vi "LVClass_WavefrontCorrector ctor.vi"(0 "WavefrontCorrector in":refnum<class "WavefrontCorrector.lvclass">, 5 "PathToWavefrontCorrectorSetupFile":path, 11 "error in (no error)":errorcluster) -> (4 "WavefrontCorrector out":refnum<class "WavefrontCorrector.lvclass">, 15 "error out":errorcluster)   [LabVIEW 2020, in "WavefrontCorrector.lvclass"]
doc: "WavefrontCorrector constructor.\n\n--------------------------------------------------------------------------------\n\n<B>correctorIn </B> : Constant Pointer to WavefrontCorrector object.\n<B>correctorOut </B> : Constant Pointer to WavefrontCorrector object.\n<B>config_file_path </B> : Absolute path to Wavefront corrector configuration file.\n<B>ErrorIn </B> : Error\n<B>ErrorOut </B> : Error\n\n--------------------------------------------------------------------------------"
uses:
  WavefrontCorrector.lvclass
  WavefrontCorrectorSet.lvclass
  Wavefront Corrector states - ONE.ctl
  WavefrontCorrector.lvclass/WavefrontCorrector.ctl
  Handle creation.ctl
  LVClass_WavefrontCorrectorSet Read AllWavefrontCorrectorParametersProperties.vi
  LVClass_WavefrontCorrectorSet Read AllWavefrontCorrectorParameters.vi
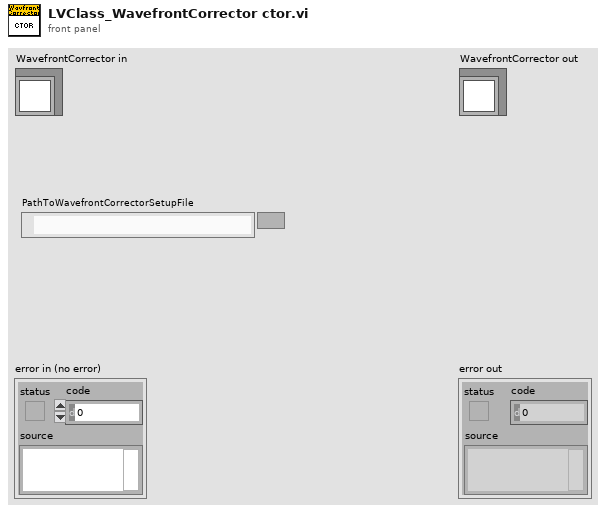
[diagram p1: front panel]
types:
  T1 = typedef "Wavefront Corrector states - ONE.ctl" = cluster{"Max":sgl, "Min":sgl, "Validity":enum16{"valid", "fixed", "invalid"}, "Fixed_Position":sgl}
  T2 = typedef "Handle creation.ctl" = enum16{"By ctor", "By write function"}
  T3 = typedef "WavefrontCorrectorSpecifications.ctl" = cluster{"Mirror name":string, "Plugin name":string, "Serial number":string, "Revision":string, "Number of commands":i32, "Sleep after command apply (ms)":i32, "Has internal memory ?":bool}
  T4 = typedef "ParameterID.ctl" = cluster{"Name":string, "Type":T5, "Authorization":T6, "OnFlyAuthorization":T7, "StringDefault":string, "Default":dbl, "Min":dbl, "Max":dbl, "Boolean":bool, "StringParameterList":string[]}
  T5 = typedef "CameraParameters_Type.ctl" = enum16{"Integer", "Real", "String", "Boolean"}
  T6 = typedef "CameraParameters_Authorization.ctl" = enum16{"Disable", "Gettable", "Settable - Gettable"}
  T7 = typedef "CameraParameters_OnFlyAuthorization.ctl" = enum16{"None", "Gettable", "Settable", "Settable - Gettable"}
  T8 = typedef "CameraParametersSetup.ctl" = cluster{"Name":string, "Type":T5, "Value":dbl, "BooleanValue":bool, "StringValue":string}
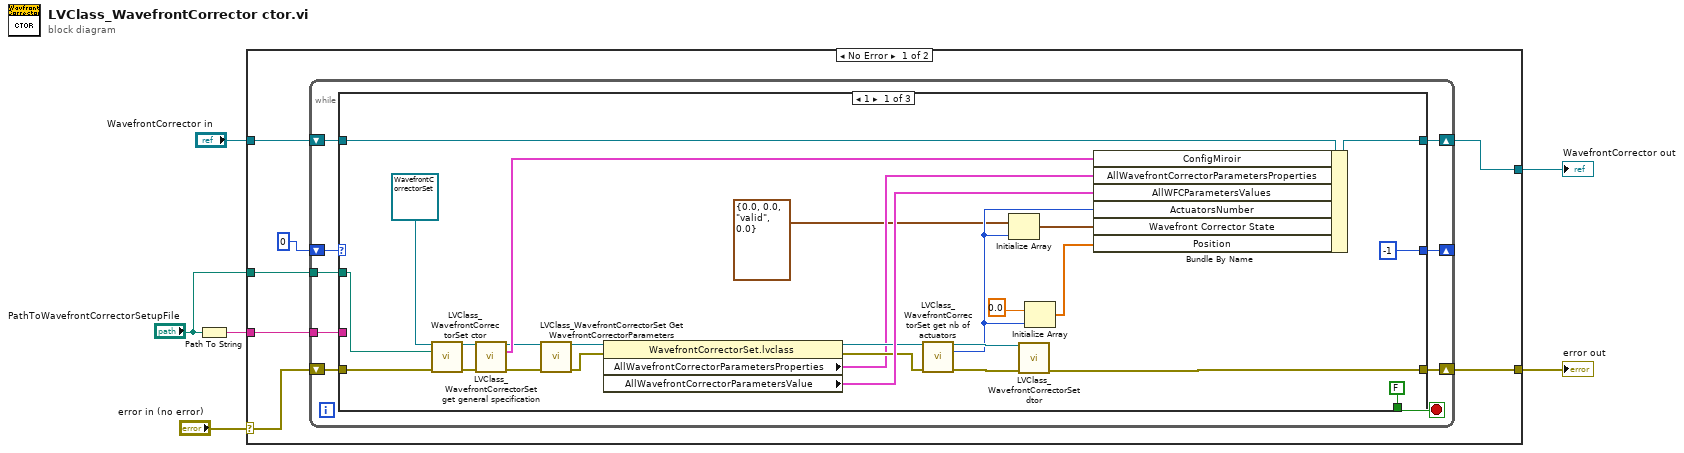
[diagram p0: block diagram]
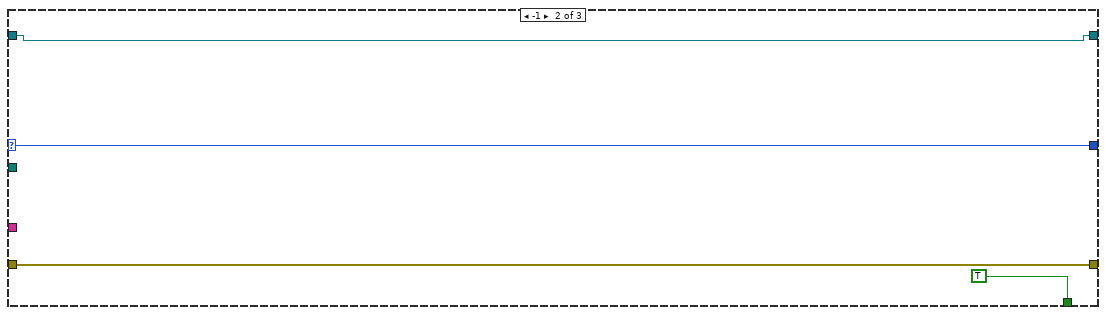
[diagram p2: hidden frame]
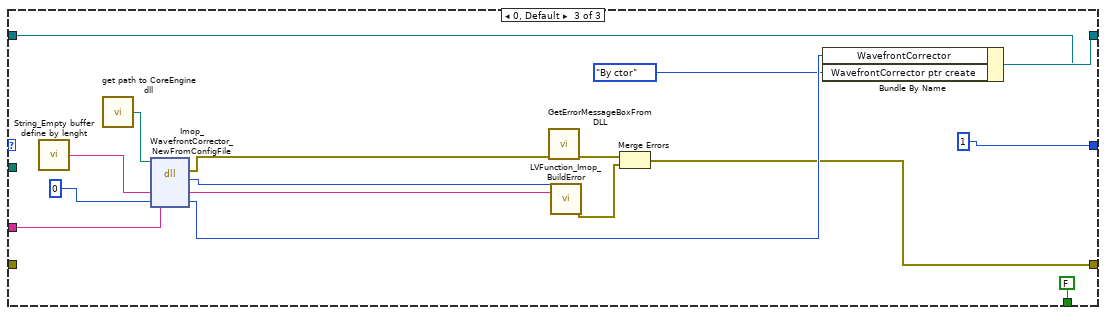
[diagram p3: hidden frame]
diagram:
  n1 = Path To String(path="PathToWavefrontCorrectorSetupFile") -> (string=w6:string)
  n2 = case shown="No Error" "error in (no error)" {
    selector: "error in (no error)" -> [w8 w70]
    tunnel: [w7 w70] -> w3
    tunnel: [w12 w69] -> w2
    tunnel: "WavefrontCorrector in" -> [w13 w69]
    tunnel: w6 -> [w11 _]
    tunnel: "PathToWavefrontCorrectorSetupFile" -> [w9 _]
    frame No Error {
      n3 = while {
        tunnel: w11 -> [w21]
        shift-right: [w19] -> _
        shift-left: 0 -> [w20]
        tunnel: w9 -> [w18]
        shift-right: [w15] -> w7
        shift-left: w8 -> [w16]
        shift-right: [w22] -> w12
        shift-left: w13 -> [w17]
        stop <- w14 stop-if-true
        n4 = case shown="1" w20 {
          selector: w20 -> [_ w52 _]
          tunnel: [w36 w49 w60] -> w22
          tunnel: [w37 w51 w57] -> w15
          tunnel: w21 -> [_ _ w56]
          tunnel: [-1 w52 1] -> w19
          tunnel: w18 -> [w46 _ _]
          tunnel: w17 -> [w45 w49 w53]
          tunnel: w16 -> [w42 w51 _]
          tunnel: [FALSE TRUE FALSE] -> w14
          frame 1 {
            n5 = call "LVClass_WavefrontCorrectorSet ctor.vi"("WavefrontCorrectorSet in"=refnum<class "WavefrontCorrectorSet.lvclass"> refnum ("WavefrontCorrectorSet.lvclass"), "PathToWavefrontCorrectorSetupFile"=w46, "error in (no error)"=w42) -> ("WavefrontCorrectorSet out"=w48:refnum<class "WavefrontCorrectorSet.lvclass">, "error out"=w43:errorcluster)  [unwired: 11 in]
            n6 = call "LVClass_WavefrontCorrectorSet get general specification.vi"("WavefrontCorrectorSet in"=w48, "error in (no error)"=w43) -> ("WavefrontCorrectorSet out"=w30:refnum<class "WavefrontCorrectorSet.lvclass">, "ConfigMiroir"=w44:T3, "error out"=w31:errorcluster)  [unwired: 11 in]
            n7 = call "LVClass_WavefrontCorrectorSet Get WavefrontCorrectorParameters.vi"("WavefrontCorrectorSet in"=w30, "error in (no error)"=w31) -> ("WavefrontCorrectorSet out"=w28:refnum<class "WavefrontCorrectorSet.lvclass">, "error out"=w26:errorcluster)  [unwired: 10 in, 2 out]
            n8 = property class="WavefrontCorrectorSet.lvclass"(reference=w28, error in=w26) -> (reference out=w27:refnum<class "WavefrontCorrectorSet.lvclass">, error out=w25:errorcluster, "AllWavefrontCorrectorParametersProperties"=w24:T4[], "AllWavefrontCorrectorParametersValue"=w29:T8[])
            n9 = call "LVClass_WavefrontCorrectorSet get nb of actuators.vi"("WavefrontCorrectorSet in"=w27, "error in (no error)"=w25) -> ("WavefrontCorrectorSet out"=w39:refnum<class "WavefrontCorrectorSet.lvclass">, "ActuatorsNumber"=w33:i32, "error out"=w38:errorcluster)  [unwired: 11 in]
            n10 = Initialize Array(T1 {"Max"=0.0, "Min"=0.0, "Validity"=enum."valid", "Fixed_Position"=0.0} ("Actuator State"), w33) -> (w35:T1[])
            n11 = call "LVClass_WavefrontCorrectorSet dtor.vi"("WavefrontCorrectorSet in"=w39, "error in (no error)"=w38) -> ("error out"=w37:errorcluster)  [unwired: 12 in, 1 out]
            n12 = Initialize Array(sgl 0.0 ("Numeric"), w33) -> (w32:sgl[])
            n13 = Bundle By Name(cluster=w45, "ConfigMiroir"=w44, "AllWavefrontCorrectorParametersProperties"=w24, "AllWFCParametersValues"=w29, "ActuatorsNumber"=w33, "Wavefront Corrector State"=w35, "Position"=w32) -> (w36:refnum<class "WavefrontCorrector.lvclass">)
          }
          frame -1 {
          }
          frame 0, Default {
            n14 = call "String_Empty buffer define by lenght.vi"() -> ("Empty buffer"=w68:string)  [unwired: 1 in]
            n15 = call "get path to CoreEngine dll.vi"() -> ("path to c_interface_vc100.dll"=w65:path)  [unwired: 12 in, 3 out]
            n16 = dll-call lib="D:/soft/HASO_v3/SVN_trunk/ImOpCoreEngine4_LV2011/DLLs/c_interface_vc100.dll" fn="Imop_WavefrontCorrector_NewFromConfigFile"(path in=w65, "message"=w68, "WavefrontCorrector"=0 ("Pupil"), "Config_file_path"=w56) -> (error out=w64:errorcluster, "return type"=w66:i32, "message"=w67:string, "WavefrontCorrector"=w62:i32)  [unwired: 3 in, 1 out]
            n17 = call "GetErrorMessageBoxFromDLL.vi"("error IN"=w64) -> ("error OUT"=w59:errorcluster)  [unwired: 10 in]
            n18 = call "LVFunction_Imop_BuildError.vi"("code"=w66, "String to Prepend to source (\"\")"=w67) -> ("error out"=w58:errorcluster)  [unwired: 13 in]
            n19 = Merge Errors(w59, w58) -> (w57:errorcluster)
            n20 = Bundle By Name(cluster=w53, "WavefrontCorrector"=w62, "WavefrontCorrector ptr create"=Handle_creation."By ctor" ("Pupil ptr create")) -> (w60:refnum<class "WavefrontCorrector.lvclass">)
          }
        }
      }
    }
    frame Error {
    }
  }
  "error out" <- w3
  "WavefrontCorrector out" <- w2
